vi "Set Routing.vi"(0 "shared in":refnum<class "niUSRP Rx Core v1 FPGA.lvclass">=refnum, 5 "routing":refnum<class "niVST Routing (Base) v1 FPGA.lvclass">=refnum) -> (4 "shared out":refnum<class "niUSRP Rx Core v1 FPGA.lvclass">)   [LabVIEW 2023]
uses:
  <instrlib>/niUSRP/Reference FPGA/Rx Core/niUSRP Rx Core v1 FPGA.lvclass
  <instrlib>/niVST/Reference FPGA/FPGA/Routing/v1/Base/niVST Routing (Base) v1 FPGA.lvclass
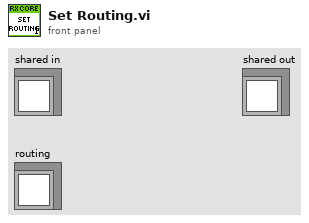
[diagram p1: front panel]
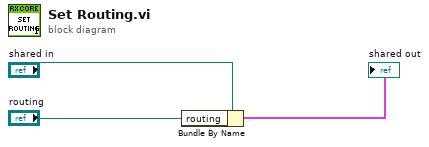
[diagram p0: block diagram]
diagram:
  n1 = Bundle By Name(cluster="shared in", "routing"="routing") -> (→"shared out":cluster{})
